vi "Pico SPI Converter (PC).vi"() -> ()   [LabVIEW 2013]
panel:
  in  "Position":i32
  in  "ConvStyle":i32
  out "element":dbl
  out "Array 4":dbl[](array[numeric])
  out "Graph":dbl[][](graph)
  in  "Numeric":i32
  in  "stop":bool
  out "Array 3":dbl[](array[numeric])
  out "Array 2":i32[](array[numeric])
  out "Array":string[](array[string])
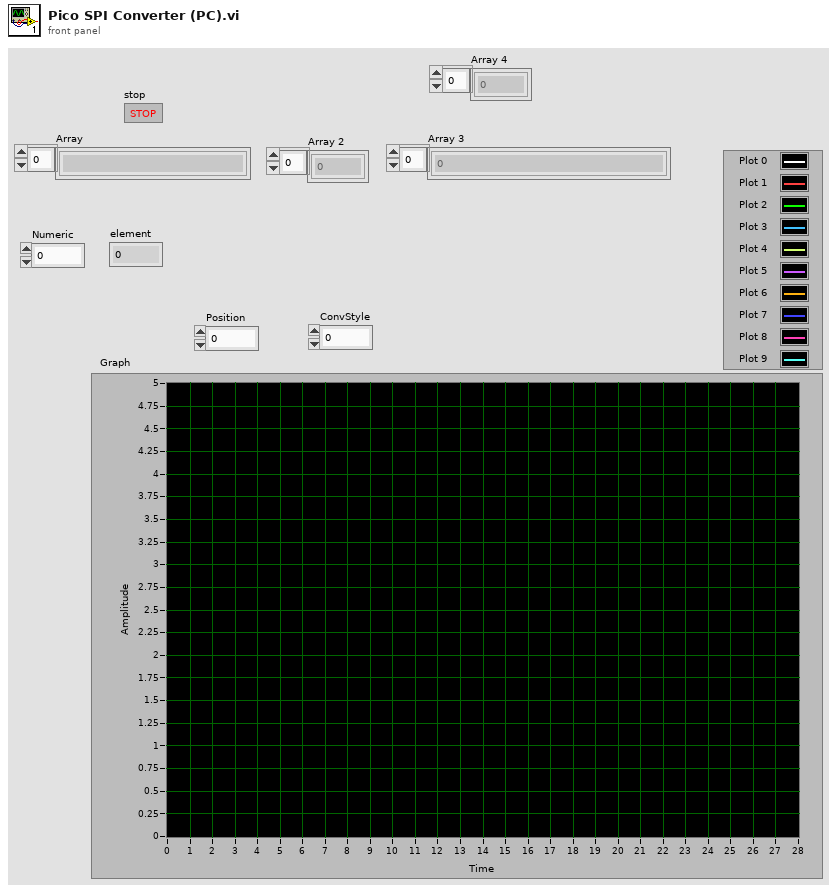
[diagram p1: front panel]
types:
  T1 = cluster{"STRstr":dbl[], "STRrev":dbl[], "REVstr":dbl[], "REVrev":dbl[]}[]
  T2 = cluster{"STRstr":dbl[], "STRrev":dbl[], "REVstr":dbl[], "REVrev":dbl[]}
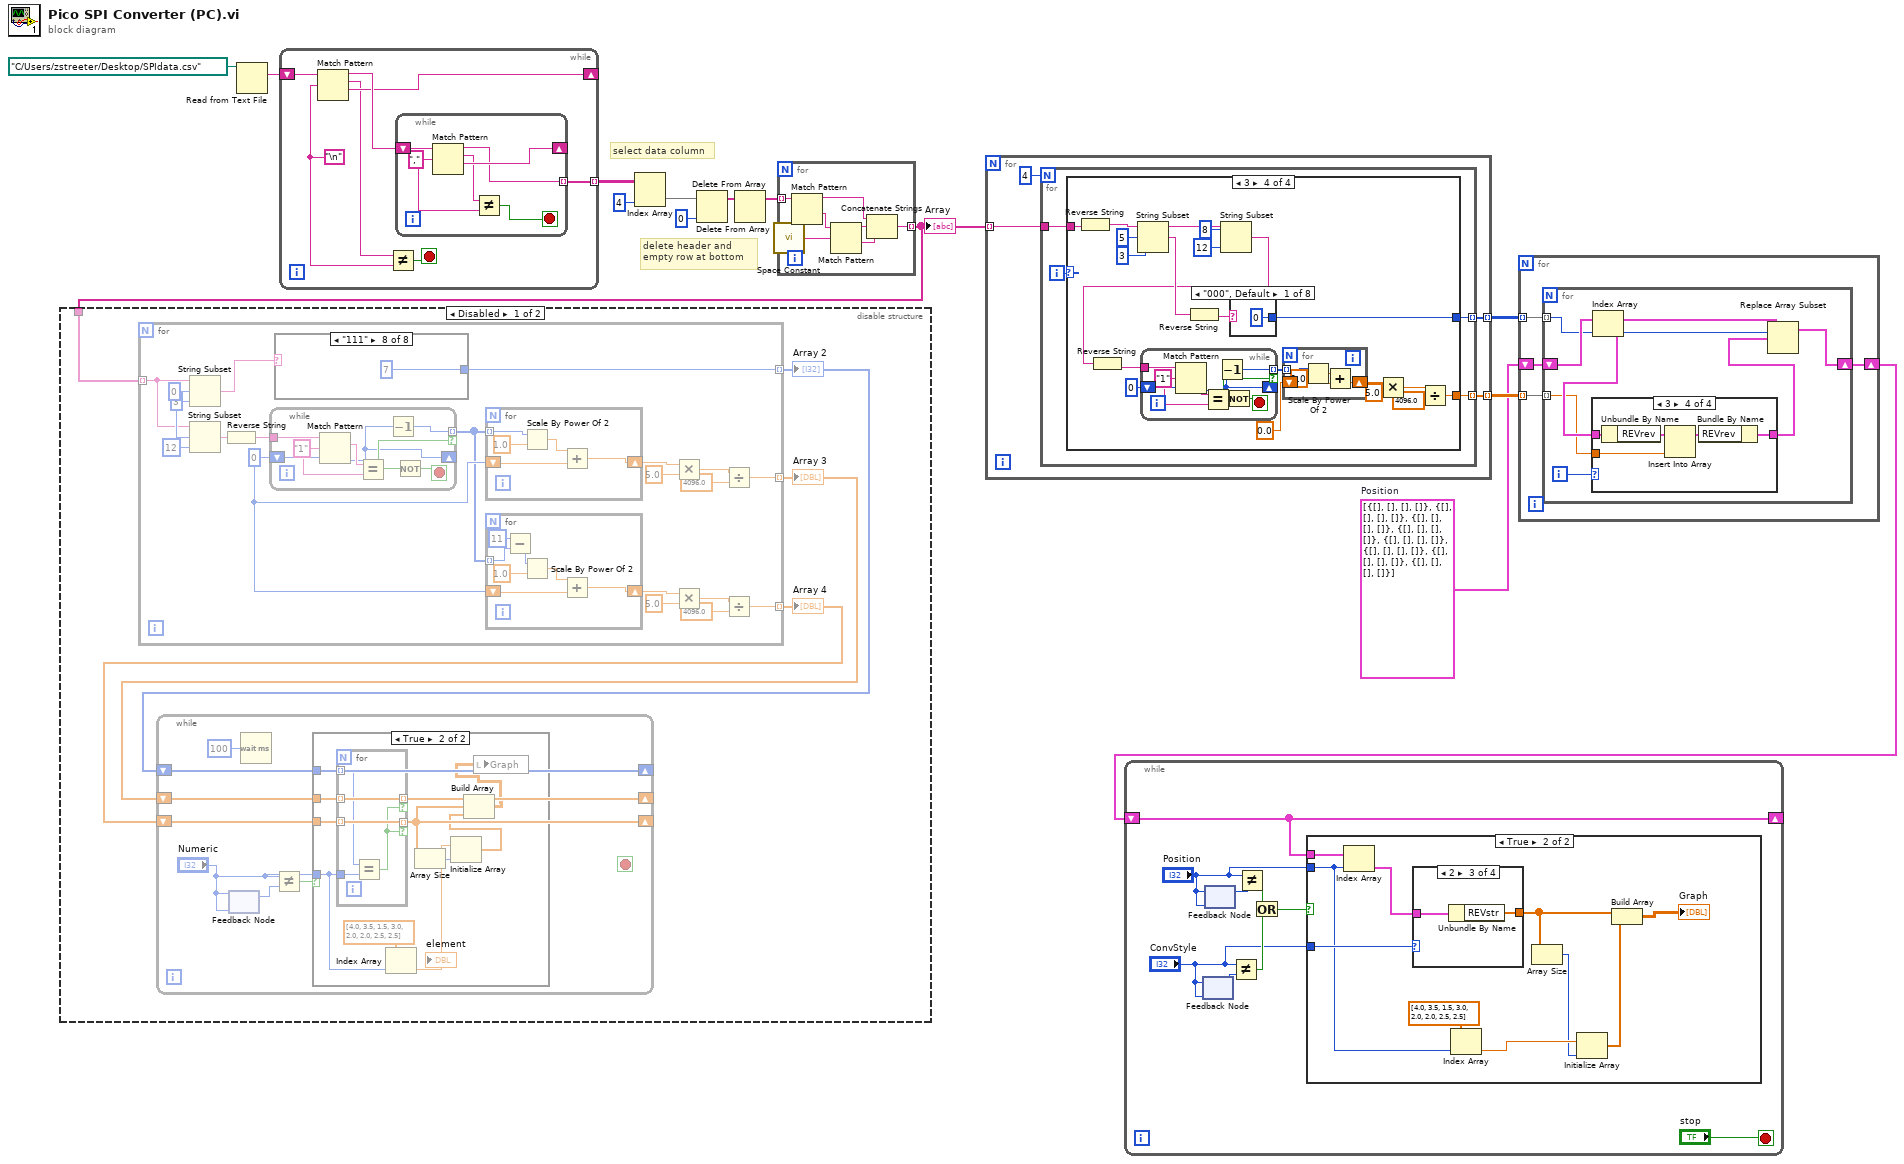
[diagram p0: block diagram]
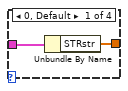
[diagram p3: hidden frame]
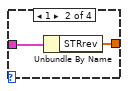
[diagram p4: hidden frame]
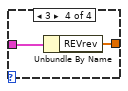
[diagram p5: hidden frame]
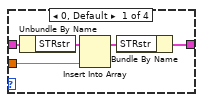
[diagram p6: hidden frame]
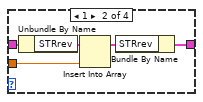
[diagram p7: hidden frame]
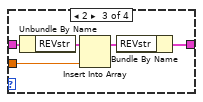
[diagram p8: hidden frame]
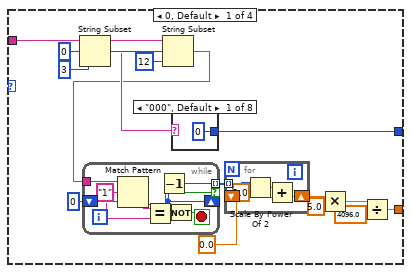
[diagram p9: hidden frame]
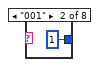
[diagram p10: hidden frame]
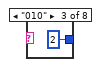
[diagram p11: hidden frame]
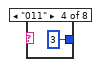
[diagram p12: hidden frame]
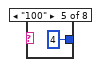
[diagram p13: hidden frame]
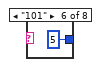
[diagram p14: hidden frame]
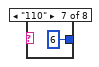
[diagram p15: hidden frame]
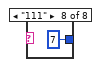
[diagram p16: hidden frame]
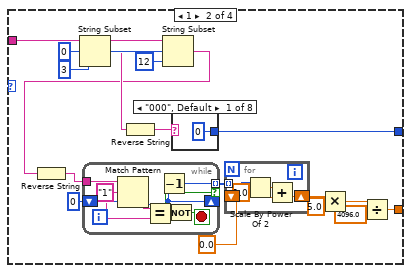
[diagram p17: hidden frame]
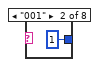
[diagram p18: hidden frame]
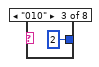
[diagram p19: hidden frame]
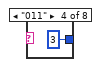
[diagram p20: hidden frame]
diagram:
  w2 = T1 [{"STRstr"=[], "STRrev"=[], "REVstr"=[], "REVrev"=[]}, {"STRstr"=[], "STRrev"=[], "REVstr"=[], "REVrev"=[]}, {"STRstr"=[], "STRrev"=[], "REVstr"=[], "REVrev"=[]}, {"STRstr"=[], "STRrev"=[], "REVstr"=[], "REVrev"=[]}, {"STRstr"=[], "STRrev"=[], "REVstr"=[], "REVrev"=[]}, {"STRstr"=[], "STRrev"=[], "REVstr"=[], "REVrev"=[]}, {"STRstr"=[], "STRrev"=[], "REVstr"=[], "REVrev"=[]}, {"STRstr"=[], "STRrev"=[], "REVstr"=[], "REVrev"=[]}]  # Position
  # "delete header and\nempty row at bottom"
  # "select data column"
  n1 = Read from Text File(file (use dialog)=path "C:/Users/zstreeter/Desktop/SPIdata.csv") -> (text=w12:string)  [unwired: 3 in, 3 out]
  n2 = while {
    shift-right: [w17] -> _
    shift-left: w12 -> [w20]
    tunnel: [w18] -> w11 mode=indexing
    stop <- w15 stop-if-true
    w14 = "\n"
    n3 = Match Pattern(string=w20, regular expression=w14) -> (before substring=w19:string, match substring=w16:string, after substring=w17:string)  [unwired: 1 in, 1 out]
    n4 = Not Equal?(x=w16, y=w14) -> (x != y?=w15:bool)
    n5 = while {
      shift-right: [w25] -> _
      shift-left: w19 -> [w26]
      tunnel: [w24] -> w18 mode=indexing
      stop <- w21 stop-if-true
      w22 = "," ("regular expression")
      n6 = Match Pattern(string=w26, regular expression=w22) -> (before substring=w24:string, match substring=w23:string, after substring=w25:string)  [unwired: 1 in, 1 out]
      n7 = Not Equal?(x=w23, y=w22) -> (x != y?=w21:bool)
    }
  }
  n8 = Index Array(array=w11, index (col)=4 ("disabled index (col)")) -> (element=w9:string[])  [unwired: 1 in]
  n9 = Delete From Array(array=w9, index=0) -> (array with subset deleted=w7:string[])  [unwired: 1 in, 1 out]
  n10 = Delete From Array(array=w7) -> (array with subset deleted=w6:string[])  [unwired: 2 in, 1 out]
  n11 = for {
    tunnel: w6 -> [w33] mode=indexing
    tunnel: [w28] -> w5 mode=indexing
    n12 = call <vilib>:"Space Constant.vi"() -> ("String"=w31:string)
    n13 = Match Pattern(string=w33, regular expression=w31) -> (before substring=w30:string, after substring=w32:string)  [unwired: 1 in, 2 out]
    n14 = Match Pattern(string=w32, regular expression=w31) -> (before substring=w29:string, after substring=w27:string)  [unwired: 1 in, 2 out]
    n15 = Concatenate Strings(w30, w29, w27) -> (w28:string)
  }
  "Array" <- w5
  n16 = disable-structure shown="Disabled" {
    disable-tunnel: w5 -> [w37 _]
    frame Disabled {
      n17 = for {
        tunnel: w37 -> [w79] mode=indexing
        tunnel: [w70] -> w35 mode=indexing
        tunnel: [w69] -> w36 mode=indexing
        tunnel: [w62] -> w34 mode=indexing
        w64 = 0 ("offset past match")
        w80 = 3 ("length (rest)")
        n18 = String Subset(string=w79, offset (0)=0, length (rest)=w80) -> (substring=w75:string)
        n19 = String Subset(string=w79, offset (0)=w80, length (rest)=12 ("length (rest)")) -> (substring=w77:string)
        n20 = Reverse String(1:w77) -> (0:w76:string)
        n21 = while {
          tunnel: w76 -> [w109]
          shift-right: [w103] -> _
          shift-left: w64 -> [w108]
          tunnel: [w102] -> w63 mode=indexing if=w105
          stop <- w104 stop-if-true
          w106 = "1" ("regular expression")
          n22 = Match Pattern(string=w109, regular expression=w106, offset (0)=w108) -> (match substring=w107:string, offset past match=w103:i32)  [unwired: 2 out]
          n23 = Equal?(x=w107, y=w106) -> (x = y?=w105:bool)
          n24 = Decrement(x=w103) -> (x-1=w102:i32)
          n25 = Not(x=w105) -> (.not. x?=w104:bool)
        }
        n26 = case shown="\"111\"" w75 {
          tunnel: [0 1 2 3 4 5 6 7] -> w69
          frame "000", Default {
          }
          frame "001" {
          }
          frame "010" {
          }
          frame "011" {
          }
          frame "100" {
          }
          frame "101" {
          }
          frame "110" {
          }
          frame "111" {
          }
        }
        n27 = for {
          tunnel: w63 -> [w100] mode=indexing
          shift-right: [w98] -> w74
          shift-left: w64 -> [w97]
          n28 = Scale By Power Of 2(n=w100, x=1.0) -> (x*2^n=w99:dbl)
          n29 = Add(x=w99, y=w97) -> (x+y=w98:dbl)
        }
        n30 = for {
          tunnel: w63 -> [w84] mode=indexing
          shift-right: [w86] -> w65
          shift-left: w64 -> [w85]
          n31 = Subtract(x=11, y=w84) -> (x-y=w82:i32)
          n32 = Scale By Power Of 2(n=w82, x=1.0) -> (x*2^n=w87:dbl)
          n33 = Add(x=w87, y=w85) -> (x+y=w86:dbl)
        }
        n34 = Multiply(x=w74, y=5.0) -> (x*y=w72:dbl)
        n35 = Multiply(x=w65, y=5.0) -> (x*y=w67:dbl)
        n36 = Divide(x=w72, y=4096.0) -> (x/y=w70:dbl)
        n37 = Divide(x=w67, y=4096.0) -> (x/y=w62:dbl)
      }
      "Array 2" <- w36
      "Array 3" <- w35
      "Array 4" <- w34
      n38 = while {
        shift-right: [w42] -> _
        shift-left: w36 -> [w42]
        shift-right: [w41] -> _
        shift-left: w35 -> [w41]
        shift-right: [w38] -> _
        shift-left: w34 -> [w38]
        stop <- w45 stop-if-true
        n39 = feedback-in #1("Numeric") -> ()
        n40 = feedback #1("Numeric") -> (w43:i32)
        n41 = Wait (ms)(milliseconds to wait=u32 100) -> ()  [unwired: 1 out]
        n42 = Not Equal?(x="Numeric", y=w43) -> (x != y?=w40:bool)
        n43 = case shown="True" w40 {
          tunnel: w42 -> [_ w56]
          tunnel: w41 -> [_ w55]
          tunnel: "Numeric" -> [_ w51]
          tunnel: w38 -> [_ w54]
          frame False {
          }
          frame True {
            n44 = for {
              tunnel: w51 -> [w60]
              tunnel: w56 -> [w61] mode=indexing
              tunnel: w55 -> [w59] mode=indexing
              tunnel: [w59] -> w53 mode=indexing if=w57
              tunnel: w54 -> [w58] mode=indexing
              tunnel: [w58] -> w50 mode=indexing if=w57
              n45 = Equal?(x=w61, y=w60) -> (x = y?=w57:bool)
            }
            n46 = Index Array(array=dbl[] [4.0, 3.5, 1.5, 3.0, 2.0, 2.0, 2.5, 2.5], index=w51) -> (element=w48:dbl)
            "element" <- w48
            n47 = Array Size(array=w50) -> (size(s)=w49:i32)
            n48 = Initialize Array(w48, w49) -> (w47:dbl[])
            n49 = Build Array(w53, w50, w47) -> (w46:dbl[][])
            n50 = local write "Graph"(w46) -> ()
          }
        }
      }
    }
    frame Enabled {
    }
  }
  n51 = for {
    tunnel: w5 -> [w112] mode=indexing
    tunnel: [w111] -> w4 mode=indexing
    tunnel: [w110] -> w3 mode=indexing
    n52 = for {
      N: 4 -> [_]
      tunnel: w112 -> [w116]
      tunnel: [w115] -> w111 mode=indexing
      tunnel: [w114] -> w110 mode=indexing
      i -> [w117]
      n53 = case shown="3" w117 {
        tunnel: w116 -> [w132 w170 w195 w237]
        tunnel: [w120 w160 w197 w239] -> w115
        tunnel: [w119 w159 w196 w238] -> w114
        frame 0, Default {
          w130 = 3 ("length (rest)")
          n54 = String Subset(string=w132, offset (0)=0, length (rest)=w130) -> (substring=w128:string)
          n55 = String Subset(string=w132, offset (0)=w130, length (rest)=12 ("length (rest)")) -> (substring=w121:string)
          n56 = while {
            tunnel: w121 -> [w145]
            shift-right: [w139] -> _
            shift-left: 0 ("offset past match") -> [w144]
            tunnel: [w138] -> w122 mode=indexing if=w141
            stop <- w140 stop-if-true
            w142 = "1" ("regular expression")
            n57 = Match Pattern(string=w145, regular expression=w142, offset (0)=w144) -> (match substring=w143:string, offset past match=w139:i32)  [unwired: 2 out]
            n58 = Equal?(x=w143, y=w142) -> (x = y?=w141:bool)
            n59 = Decrement(x=w139) -> (x-1=w138:i32)
            n60 = Not(x=w141) -> (.not. x?=w140:bool)
          }
          n61 = case shown="\"000\", Default" w128 {
            tunnel: [0 1 2 3 4 5 6 7] -> w120
            frame "000", Default {
            }
            frame "001" {
            }
            frame "010" {
            }
            frame "011" {
            }
            frame "100" {
            }
            frame "101" {
            }
            frame "110" {
            }
            frame "111" {
            }
          }
          n62 = for {
            tunnel: w122 -> [w136] mode=indexing
            shift-right: [w134] -> w127
            shift-left: 0.0 -> [w133]
            n63 = Scale By Power Of 2(n=w136, x=1.0) -> (x*2^n=w135:dbl)
            n64 = Add(x=w135, y=w133) -> (x+y=w134:dbl)
          }
          n65 = Multiply(x=w127, y=5.0) -> (x*y=w125:dbl)
          n66 = Divide(x=w125, y=4096.0) -> (x/y=w119:dbl)
        }
        frame 1 {
          w168 = 3 ("length (rest)")
          n67 = String Subset(string=w170, offset (0)=0, length (rest)=w168) -> (substring=w158:string)
          n68 = Reverse String(1:w158) -> (0:w156:string)
          n69 = String Subset(string=w170, offset (0)=w168, length (rest)=12 ("length (rest)")) -> (substring=w157:string)
          n70 = Reverse String(1:w157) -> (0:w155:string)
          n71 = while {
            tunnel: w155 -> [w183]
            shift-right: [w177] -> _
            shift-left: 0 ("offset past match") -> [w182]
            tunnel: [w176] -> w161 mode=indexing if=w179
            stop <- w178 stop-if-true
            w180 = "1" ("regular expression")
            n72 = Match Pattern(string=w183, regular expression=w180, offset (0)=w182) -> (match substring=w181:string, offset past match=w177:i32)  [unwired: 2 out]
            n73 = Equal?(x=w181, y=w180) -> (x = y?=w179:bool)
            n74 = Decrement(x=w177) -> (x-1=w176:i32)
            n75 = Not(x=w179) -> (.not. x?=w178:bool)
          }
          n76 = case shown="\"000\", Default" w156 {
            tunnel: [0 1 2 3 4 5 6 7] -> w160
            frame "000", Default {
            }
            frame "001" {
            }
            frame "010" {
            }
            frame "011" {
            }
            frame "100" {
            }
            frame "101" {
            }
            frame "110" {
            }
            frame "111" {
            }
          }
          n77 = for {
            tunnel: w161 -> [w174] mode=indexing
            shift-right: [w172] -> w166
            shift-left: 0.0 -> [w171]
            n78 = Scale By Power Of 2(n=w174, x=1.0) -> (x*2^n=w173:dbl)
            n79 = Add(x=w173, y=w171) -> (x+y=w172:dbl)
          }
          n80 = Multiply(x=w166, y=5.0) -> (x*y=w164:dbl)
          n81 = Divide(x=w164, y=4096.0) -> (x/y=w159:dbl)
        }
        frame 2 {
          n82 = Reverse String(1:w195) -> (0:w194:string)
          n83 = String Subset(string=w194, offset (0)=5, length (rest)=3 ("length (rest)")) -> (substring=w205:string)
          n84 = String Subset(string=w194, offset (0)=8, length (rest)=12 ("length (rest)")) -> (substring=w198:string)
          n85 = while {
            tunnel: w198 -> [w221]
            shift-right: [w215] -> _
            shift-left: 0 ("offset past match") -> [w220]
            tunnel: [w214] -> w199 mode=indexing if=w217
            stop <- w216 stop-if-true
            w218 = "1" ("regular expression")
            n86 = Match Pattern(string=w221, regular expression=w218, offset (0)=w220) -> (match substring=w219:string, offset past match=w215:i32)  [unwired: 2 out]
            n87 = Equal?(x=w219, y=w218) -> (x = y?=w217:bool)
            n88 = Decrement(x=w215) -> (x-1=w214:i32)
            n89 = Not(x=w217) -> (.not. x?=w216:bool)
          }
          n90 = case shown="\"000\", Default" w205 {
            tunnel: [0 1 2 3 4 5 6 7] -> w197
            frame "000", Default {
            }
            frame "001" {
            }
            frame "010" {
            }
            frame "011" {
            }
            frame "100" {
            }
            frame "101" {
            }
            frame "110" {
            }
            frame "111" {
            }
          }
          n91 = for {
            tunnel: w199 -> [w212] mode=indexing
            shift-right: [w210] -> w204
            shift-left: 0.0 -> [w209]
            n92 = Scale By Power Of 2(n=w212, x=1.0) -> (x*2^n=w211:dbl)
            n93 = Add(x=w211, y=w209) -> (x+y=w210:dbl)
          }
          n94 = Multiply(x=w204, y=5.0) -> (x*y=w202:dbl)
          n95 = Divide(x=w202, y=4096.0) -> (x/y=w196:dbl)
        }
        frame 3 {
          n96 = Reverse String(1:w237) -> (0:w236:string)
          n97 = String Subset(string=w236, offset (0)=5, length (rest)=3 ("length (rest)")) -> (substring=w235:string)
          n98 = Reverse String(1:w235) -> (0:w234:string)
          n99 = String Subset(string=w236, offset (0)=8, length (rest)=12 ("length (rest)")) -> (substring=w233:string)
          n100 = Reverse String(1:w233) -> (0:w232:string)
          n101 = while {
            tunnel: w232 -> [w261]
            shift-right: [w255] -> _
            shift-left: 0 ("offset past match") -> [w260]
            tunnel: [w254] -> w240 mode=indexing if=w257
            stop <- w256 stop-if-true
            w258 = "1" ("regular expression")
            n102 = Match Pattern(string=w261, regular expression=w258, offset (0)=w260) -> (match substring=w259:string, offset past match=w255:i32)  [unwired: 2 out]
            n103 = Equal?(x=w259, y=w258) -> (x = y?=w257:bool)
            n104 = Decrement(x=w255) -> (x-1=w254:i32)
            n105 = Not(x=w257) -> (.not. x?=w256:bool)
          }
          n106 = case shown="\"000\", Default" w234 {
            tunnel: [0 1 2 3 4 5 6 7] -> w239
            frame "000", Default {
            }
            frame "001" {
            }
            frame "010" {
            }
            frame "011" {
            }
            frame "100" {
            }
            frame "101" {
            }
            frame "110" {
            }
            frame "111" {
            }
          }
          n107 = for {
            tunnel: w240 -> [w252] mode=indexing
            shift-right: [w250] -> w245
            shift-left: 0.0 -> [w249]
            n108 = Scale By Power Of 2(n=w252, x=1.0) -> (x*2^n=w251:dbl)
            n109 = Add(x=w251, y=w249) -> (x+y=w250:dbl)
          }
          n110 = Multiply(x=w245, y=5.0) -> (x*y=w243:dbl)
          n111 = Divide(x=w243, y=4096.0) -> (x/y=w238:dbl)
        }
      }
    }
  }
  n112 = for {
    tunnel: w4 -> [w273] mode=indexing
    tunnel: w3 -> [w270] mode=indexing
    shift-right: [w271] -> w1
    shift-left: w2 -> [w272]
    n113 = for {
      tunnel: w273 -> [w279] mode=indexing
      shift-right: [w274] -> w271
      shift-left: w272 -> [w280]
      tunnel: w270 -> [w276] mode=indexing
      i -> [w278]
      n114 = Index Array(array=w280, index=w279) -> (element=w277:T2)
      n115 = case shown="3" w278 {
        tunnel: w277 -> [w285 w290 w295 w300]
        tunnel: w276 -> [w281 w286 w291 w296]
        tunnel: [w282 w287 w292 w297] -> w275
        frame 0, Default {
          n116 = Unbundle By Name(w285) -> ("STRstr"=w284:dbl[])
          n117 = Insert Into Array(array=w284, new element=w281) -> (w283:dbl[])  [unwired: 1 in]
          n118 = Bundle By Name(cluster=w285, "STRstr"=w283) -> (w282:T2)
        }
        frame 1 {
          n119 = Unbundle By Name(w290) -> ("STRrev"=w289:dbl[])
          n120 = Insert Into Array(array=w289, new element=w286) -> (w288:dbl[])  [unwired: 1 in]
          n121 = Bundle By Name(cluster=w290, "STRrev"=w288) -> (w287:T2)
        }
        frame 2 {
          n122 = Unbundle By Name(w295) -> ("REVstr"=w294:dbl[])
          n123 = Insert Into Array(array=w294, new element=w291) -> (w293:dbl[])  [unwired: 1 in]
          n124 = Bundle By Name(cluster=w295, "REVstr"=w293) -> (w292:T2)
        }
        frame 3 {
          n125 = Unbundle By Name(w300) -> ("REVrev"=w299:dbl[])
          n126 = Insert Into Array(array=w299, new element=w296) -> (w298:dbl[])  [unwired: 1 in]
          n127 = Bundle By Name(cluster=w300, "REVrev"=w298) -> (w297:T2)
        }
      }
      n128 = Replace Array Subset(array=w280, new element=w275, index=w279) -> (w274:T1)
    }
  }
  n129 = while {
    shift-right: [w304] -> _
    shift-left: w1 -> [w304]
    stop <- "stop" stop-if-true
    n130 = feedback #2("ConvStyle") -> (w308:i32)
    n131 = feedback-in #2("ConvStyle") -> ()
    n132 = feedback-in #3("Position") -> ()
    n133 = feedback #3("Position") -> (w309:i32)
    n134 = Not Equal?(x="ConvStyle", y=w308) -> (x != y?=w306:bool)
    n135 = Not Equal?(x="Position", y=w309) -> (x != y?=w307:bool)
    n136 = Or(x=w307, y=w306) -> (x .or. y?=w303:bool)
    n137 = case shown="True" w303 {
      tunnel: w304 -> [_ w319]
      tunnel: "Position" -> [_ w315]
      tunnel: "ConvStyle" -> [_ w318]
      frame False {
      }
      frame True {
        n138 = Index Array(array=w319, index=w315) -> (element=w317:T2)
        n139 = case shown="2" w318 {
          tunnel: w317 -> [w321 w323 w325 w327]
          tunnel: [w320 w322 w324 w326] -> w311
          frame 0, Default {
            n140 = Unbundle By Name(w321) -> ("STRstr"=w320:dbl[])
          }
          frame 1 {
            n141 = Unbundle By Name(w323) -> ("STRrev"=w322:dbl[])
          }
          frame 2 {
            n142 = Unbundle By Name(w325) -> ("REVstr"=w324:dbl[])
          }
          frame 3 {
            n143 = Unbundle By Name(w327) -> ("REVrev"=w326:dbl[])
          }
        }
        n144 = Index Array(array=dbl[] [4.0, 3.5, 1.5, 3.0, 2.0, 2.0, 2.5, 2.5], index=w315) -> (element=w314:dbl)
        n145 = Array Size(array=w311) -> (size(s)=w313:i32)
        n146 = Initialize Array(w314, w313) -> (w312:dbl[])
        n147 = Build Array(w311, w312) -> (→"Graph":dbl[][])
      }
    }
  }
